vi "Write ADU Packet.vi"(8 "error in":errorcluster, 9 "SMSD Data Unit":refnum<class "SMSD Data Unit.lvclass">, 10 "isMaster (f)":bool, 11 "IP simple ADU in":refnum<class "SMSD ADU.lvclass">) -> (0 "error out":errorcluster, 3 "IP simple ADU out":refnum<class "SMSD ADU.lvclass">)   [LabVIEW 2021, in "SMSD ADU.lvclass"]
doc: "This uses the protocol layer to write a modbus packet to the bus, wrapped in the IP transmission data unit."
uses:
  SMSD ADU.lvclass
  Data Unit/SMSD Data Unit/SMSD Data Unit.lvclass
  SMSD ADU.lvclass/SMSD ADU.ctl
  Data Unit/SMSD Data Unit/SMSD Data Unit.lvclass/SMSD Data Unit.ctl
  <vilib>/Utility/error.llb/Clear Errors.vi
  Modbus_v121c/Network Interface/TCP Interface/TCP Shared Components/TCP Shared Components.lvlib
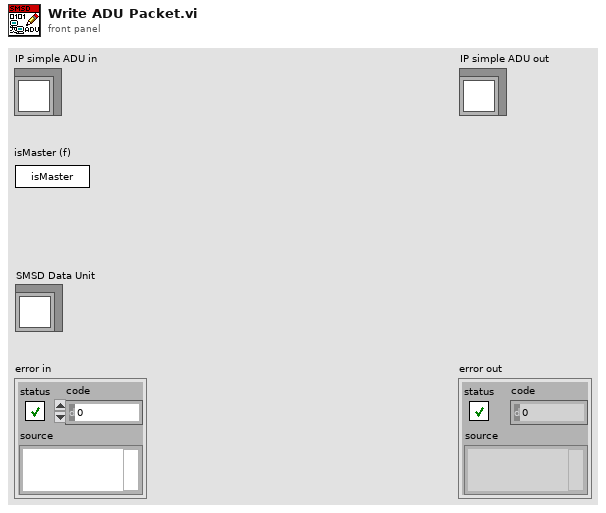
[diagram p1: front panel]
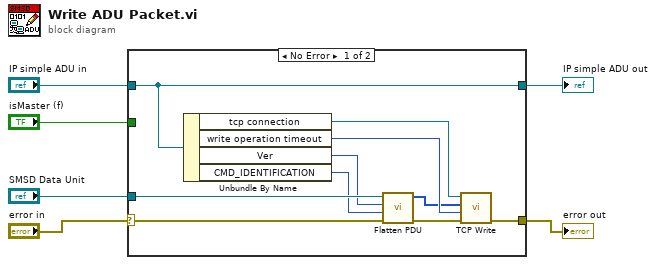
[diagram p0: block diagram]
diagram:
  n1 = case shown="No Error" "error in" {
    selector: "error in" -> [w9 w17]
    tunnel: [w15 w17] -> w3
    tunnel: "IP simple ADU in" -> [w14 w18]
    tunnel: [w14 w18] -> w5
    tunnel: "isMaster (f)" -> [_ _]
    tunnel: "SMSD Data Unit" -> [w12 _]
    frame No Error {
      n2 = Unbundle By Name(w14) -> ("tcp connection"=w16:refnum<k5>, "write operation timeout"=w13:u32, "Ver"=w11:u8, "CMD_IDENTIFICATION"=w7:u8)
      n3 = call "Flatten PDU.vi"("error in"=w9, "CMD_IDENTIFICATION"=w7, "Ver"=w11, "SMSD data unit in"=w12) -> ("error out"=w8:errorcluster, "Full SMSD data unit"=w10:u8[])  [unwired: 6 in]
      n4 = call "TCP Write.vi"("error in"=w8, "timeout"=w13, "data"=w10, "connection ID"=w16) -> ("error out"=w15:errorcluster)  [unwired: 6 in, 1 out]
    }
    frame Error {
    }
  }
  "error out" <- w3
  "IP simple ADU out" <- w5
